vi "Teleop.vi"(10 "Match Info":T1={"Autonomous Elapsed Seconds"=0.0, "TeleOp Elapsed Seconds"=0.0, "Disabled Elapsed Seconds"=0.0, "Visited Autonomous"=FALSE, "Visited TeleOp"=FALSE, "Visited Disabled"=FALSE, "Autonomous Settings"={"Autonomous Style"=enum."Independent", "VI Refnum"=refnum}}, 11 "Call Context":T2) -> ()   [LabVIEW 2017]
doc: "This VI is called for each TeleOp packet received from the DS where the robot is not disabled. It is often used to read from the joysticks and update I/O or to update setpoints for timed control loops. It should complete and return within 20 milliseconds or it may miss DS packets."
uses:
  <vilib>/Rock Robotics/WPI/DriverStation/WPI_DriverStationDerivedRobotMode.ctl
  <vilib>/Rock Robotics/WPI/DriverStation/WPI_DriverStationMatch Info.ctl
  <vilib>/Rock Robotics/WPI/Utilities/WPI_GetSetVariantRefNum.vi
  <vilib>/Rock Robotics/Network Tables/NT Write Boolean Array.vi
  <vilib>/Rock Robotics/Network Tables/NT Write Numeric Array.vi
  <vilib>/Rock Robotics/Network Tables/NT Read Boolean.vi
  <vilib>/Rock Robotics/Network Tables/NT Read Number.vi
panel:
  out "Sample Slider 0":dbl(slide) scale=0.0..5.0
  out "Sample Boolean 1":bool
  out "Sample Boolean 0":bool
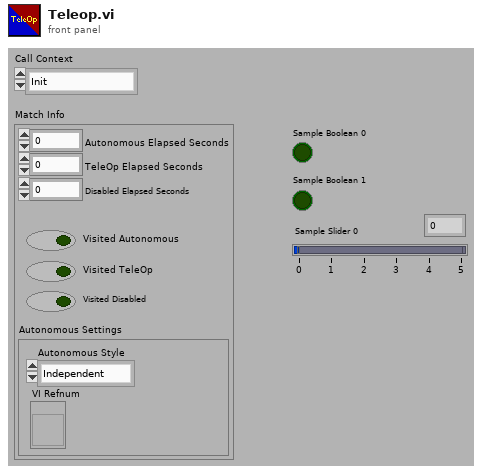
[diagram p1: front panel]
types:
  T1 = typedef "WPI_DriverStationMatch Info.ctl" = cluster{"Autonomous Elapsed Seconds":dbl, "TeleOp Elapsed Seconds":dbl, "Disabled Elapsed Seconds":dbl, "Visited Autonomous":bool, "Visited TeleOp":bool, "Visited Disabled":bool, "Autonomous Settings":cluster{"Autonomous Style":enum16{"Iterative", "Independent"}, "VI Refnum":refnum<vi>}}
  T2 = typedef "WPI_DriverStationDerivedRobotMode.ctl" = enum16{"Init", "Execute", "Stop"}
  T3 = typedef "WPI_JoystickDevRef.ctl" = cluster{"Device":T4}
  T4 = typedef "WPI_JoystickDeviceEnum.ctl" = enum16{"USB 0", "USB 1", "USB 2", "USB 3", "USB 4", "USB 5"}
  T5 = cluster{"Buttons[0]":bool, "Buttons[1]":bool, "Buttons[2]":bool, "Buttons[3]":bool, "Buttons[4]":bool, "Buttons[5]":bool, "Buttons[6]":bool, "Buttons[7]":bool, "Buttons[8]":bool}
  T6 = cluster{"Axes[0]":dbl, "Axes[1]":dbl, "Axes[2]":dbl, "Axes[3]":dbl, "Axes[4]":dbl, "Axes[5]":dbl, "Axes[6]":dbl, "Axes[7]":dbl, "Axes[8]":dbl}
  T7 = typedef "WPI_MotorControlDeviceRef.ctl" = cluster{"DeviceStatus":errorcluster, "Type":T8, "PWM":cluster{"PWM Channel":T9, "DeadBand":T10}, "CAN":cluster{"Device Number":u8, "SetOutput VI Ref":variant, "GetOutput VI Ref":variant, "Enable VI Ref":variant, "Disable VI Ref":variant, "Data":variant}, "Invert":bool, "DIO PWM":cluster{"PWM \"Enable\" Channel":T9, "DIOChannel":T11, "PWM Rate":dbl}}
  T8 = typedef "WPI_MotorControlType.ctl" = enum16{"PWM", "CAN", "DIO PWM"}
  T9 = typedef "FPGA_DIOPWMChannel.ctl" = enum8{"PWM 0", "PWM 1", "PWM 2", "PWM 3", "PWM 4", "PWM 5", "PWM 6", "PWM 7", "PWM 8", "PWM 9", "PWM MXP 0", "PWM MXP 1", "PWM MXP 2", "PWM MXP 3", "PWM MXP 4", "PWM MXP 5", "PWM MXP 6", "PWM MXP 7", "PWM MXP 8", "PWM MXP 9", "Invalid"}
  T10 = typedef "WPI_PWMDeadband.ctl" = cluster{"Name":string, "maxPositivePwm":i32, "minPositivePwm":i32, "centerPwm":i32, "maxNegativePwm":i32, "minNegativePwm":i32, "angularRange":u16}
  T11 = typedef "FPGA_DIOChannel.ctl" = enum8{"DIO 0", "DIO 1", "DIO 2", "DIO 3", "DIO 4", "DIO 5", "DIO 6", "DIO 7", "DIO 8", "DIO 9", "DIO MXP 0", "DIO MXP 1", "DIO MXP 2", "DIO MXP 3", "DIO MXP 4", "DIO MXP 5", "DIO MXP 6", "DIO MXP 7", "DIO MXP 8", "DIO MXP 9", "DIO MXP 10", "DIO MXP 11", "DIO MXP 12", "DIO MXP 13", "DIO MXP 14", "DIO MXP 15", "SPI Port CS1", "SPI Port CS2", "SPI Port CS3", "SPI Port MISO", "SPI Port MOSI", "Invalid"}
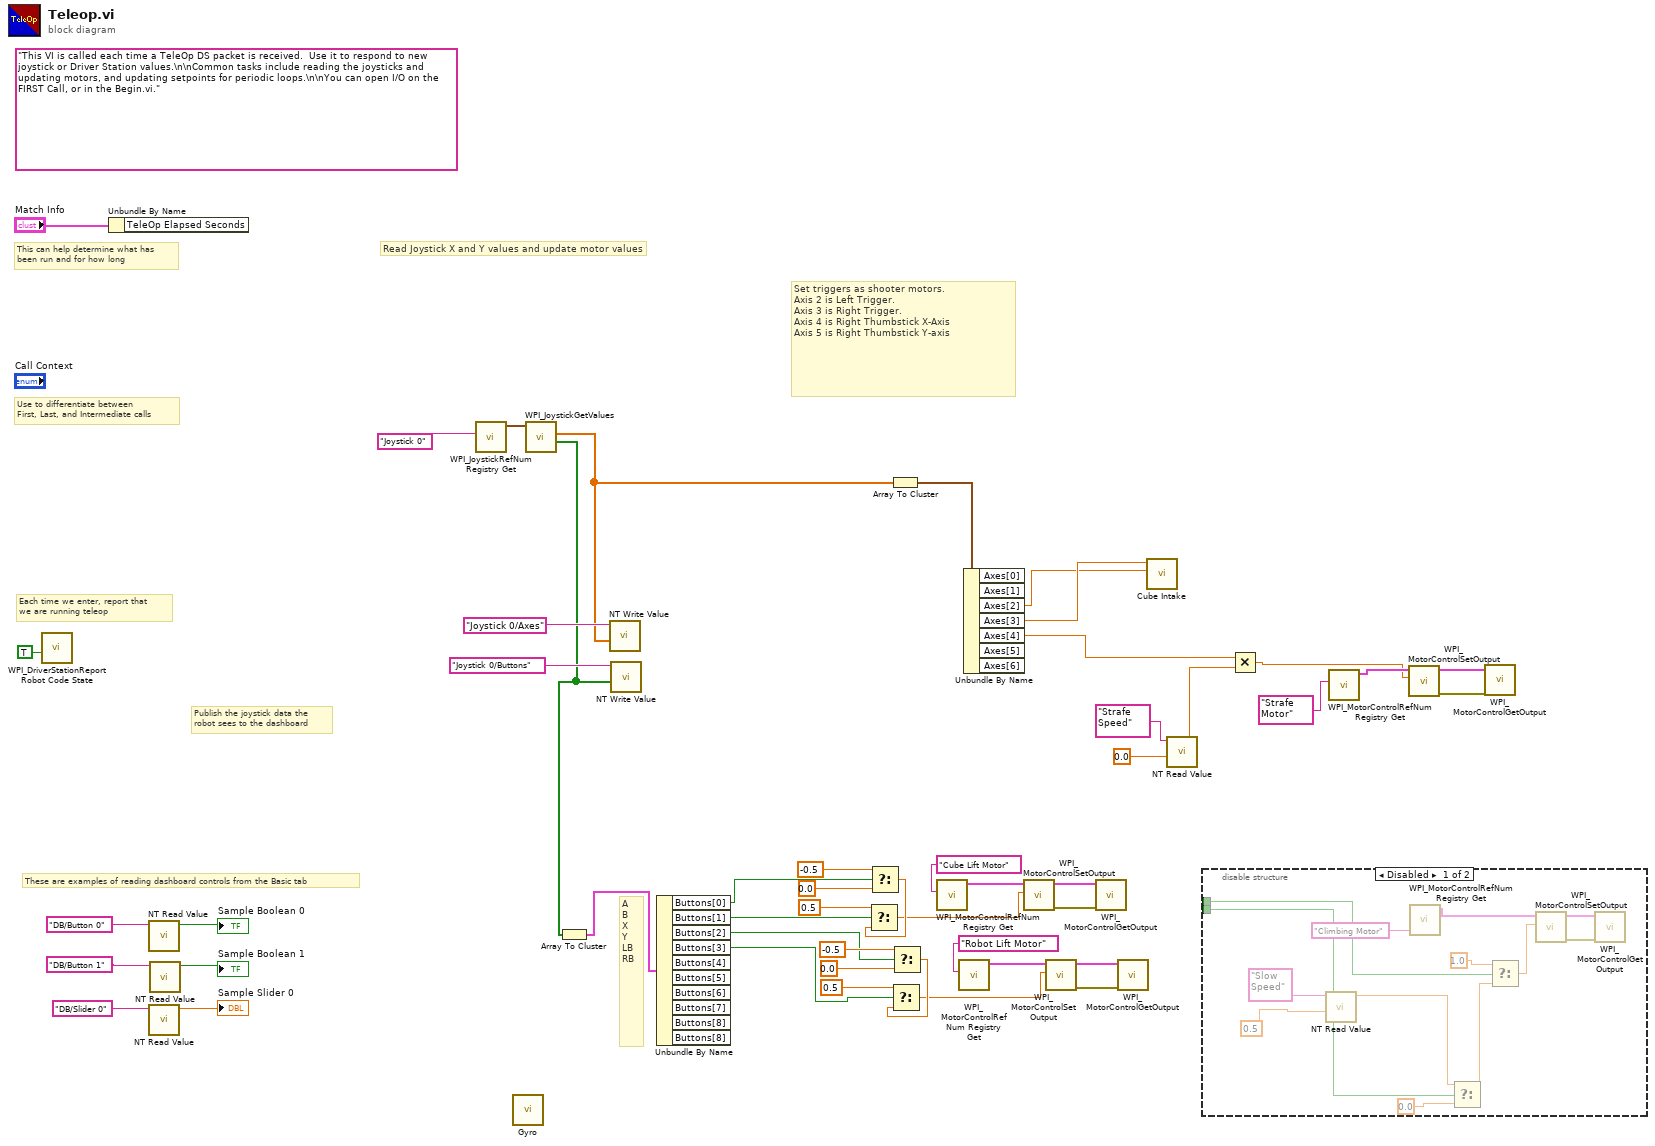
[diagram p0: block diagram]
diagram:
  (unwired) "This VI is called each time a TeleOp DS packet is received.  Use it to respond to new joystick or Driver Station values.\n\nCommon tasks include reading the joysticks and updating motors, and updating setpoints for periodic loops.\n\nYou can open I/O on the FIRST Call, or in the Begin.vi."
  # "Set triggers as shooter motors.  \nAxis 2 is Left Trigger.  \nAxis 3 is Right Trigger.\nAxis 4 is Right Thumbstick X-Axis\nAxis 5 is Right Thumbstick Y-axis"
  # "A\nB\nX\nY\nLB\nRB"
  # "These are examples of reading dashboard controls from the Basic tab"
  # "Publish the joystick data the\nrobot sees to the dashboard"
  # "Each time we enter, report that\nwe are running teleop"
  # "Use to differentiate between\nFirst, Last, and Intermediate calls"
  # "This can help determine what has\nbeen run and for how long"
  # "Read Joystick X and Y values and update motor values"
  n1 = call <vilib>:"WPI_DriverStationReport Robot Code State.vi"("TeleOp"=TRUE ("Autonomous")) -> ()  [unwired: 10 in, 1 out]
  n2 = Unbundle By Name("Match Info") -> ()  [unwired: 1 out]
  n3 = call-poly <vilib>:"NT Read Value.vi"("Name"="DB/Button 0" ("refnum name")) -> ("Boolean"=→"Sample Boolean 0":bool)  [unwired: 9 in, 1 out]
  n4 = call-poly <vilib>:"NT Read Value.vi"("Name"="DB/Slider 0" ("refnum name")) -> ("Numeric"=→"Sample Slider 0":dbl)  [unwired: 9 in, 1 out]
  n5 = call-poly <vilib>:"NT Read Value.vi"("Name"="DB/Button 1" ("refnum name")) -> ("Boolean"=→"Sample Boolean 1":bool)  [unwired: 9 in, 1 out]
  n6 = call <vilib>:"WPI_JoystickRefNum Registry Get.vi"("refnum name"="Joystick 0") -> ("JoystickDevRef"=w47:T3)  [unwired: 1 in, 9 out]
  n7 = call "Gyro.vi"() -> ()  [unwired: 12 in]
  n8 = call <vilib>:"WPI_JoystickGetValues.vi"("JoystickDevRef"=w47) -> ("Buttons"=w37:bool[], "Axes"=w35:dbl[])  [unwired: 6 in, 3 out]
  n9 = Array To Cluster(array=w37) -> (cluster=w18:T5)
  n10 = call-poly <vilib>:"NT Write Value.vi"("Numeric Array"=w35, "Name"="Joystick 0/Axes") -> ()  [unwired: 9 in, 1 out]
  n11 = call-poly <vilib>:"NT Write Value.vi"("Boolean Array"=w37, "Name"="Joystick 0/Buttons") -> ()  [unwired: 9 in, 1 out]
  n12 = Unbundle By Name(w18) -> ("Buttons[0]"=w15:bool, "Buttons[1]"=w17:bool, "Buttons[2]"=w2:bool, "Buttons[3]"=w1:bool)  [unwired: 6 out]
  n13 = Select(t=-0.5, s=w15, f=0.0) -> (s? t:f=w13:dbl)
  n14 = Select(t=0.5, s=w17, f=w13) -> (s? t:f=w12:dbl)
  n15 = Array To Cluster(array=w35) -> (cluster=w36:T6)
  n16 = Select(t=-0.5, s=w2, f=0.0) -> (s? t:f=w4:dbl)
  n17 = Select(t=0.5, s=w1, f=w4) -> (s? t:f=w3:dbl)
  n18 = call <vilib>:"WPI_MotorControlRefNum Registry Get.vi"("refnum name"="Cube Lift Motor") -> ("MotorControlDevRef"=w21:T7)  [unwired: 9 in, 1 out]
  n19 = call <vilib>:"WPI_MotorControlRefNum Registry Get.vi"("refnum name"="Robot Lift Motor") -> ("MotorControlDevRef"=w9:T7)  [unwired: 9 in, 1 out]
  n20 = Unbundle By Name(w36) -> ("Axes[2]"=w32:dbl, "Axes[3]"=w33:dbl, "Axes[4]"=w34:dbl)  [unwired: 4 out]
  n21 = call <vilib>:"WPI_MotorControlSetOutput.vi"("Output"=w12, "MotorControlDevRef"=w21) -> ("error out"=w23:errorcluster, "MotorControlDevRef"=w22:T7)  [unwired: 7 in, 1 out]
  n22 = call <vilib>:"WPI_MotorControlSetOutput.vi"("Output"=w3, "MotorControlDevRef"=w9) -> ("error out"=w11:errorcluster, "MotorControlDevRef"=w10:T7)  [unwired: 7 in, 1 out]
  n23 = call <vilib>:"WPI_MotorControlGetOutput.vi"("error in"=w23, "MotorControlDevRef"=w22) -> ()  [unwired: 7 in, 3 out]
  n24 = call <vilib>:"WPI_MotorControlGetOutput.vi"("error in"=w11, "MotorControlDevRef"=w10) -> ()  [unwired: 7 in, 3 out]
  n25 = call "Cube Intake.vi"("Axes[2]"=w32, "Axes[3]"=w33) -> ()  [unwired: 10 in]
  n26 = call-poly <vilib>:"NT Read Value.vi"("Default Value"=0.0, "Name"="Strafe Speed") -> ("Numeric"=w25:dbl)  [unwired: 8 in, 1 out]
  n27 = disable-structure shown="Disabled" {
    disable-tunnel: _ -> [w51 _]
    disable-tunnel: _ -> [w50 _]
    frame Disabled {
      n28 = call-poly <vilib>:"NT Read Value.vi"("Default Value"=0.5, "Name"="Slow Speed" ("refnum name")) -> ("Numeric"=w54:dbl)  [unwired: 8 in, 1 out]
      n29 = call <vilib>:"WPI_MotorControlRefNum Registry Get.vi"("refnum name"="Climbing Motor") -> ("MotorControlDevRef"=w53:T7)  [unwired: 9 in, 1 out]
      n30 = Select(t=w54, s=w50, f=0.0) -> (s? t:f=w57:dbl)
      n31 = Select(t=1.0, s=w51, f=w57) -> (s? t:f=w59:dbl)
      n32 = call <vilib>:"WPI_MotorControlSetOutput.vi"("Output"=w59, "MotorControlDevRef"=w53) -> ("error out"=w61:errorcluster, "MotorControlDevRef"=w62:T7)  [unwired: 7 in, 1 out]
      n33 = call <vilib>:"WPI_MotorControlGetOutput.vi"("error in"=w61, "MotorControlDevRef"=w62) -> ()  [unwired: 7 in, 3 out]
    }
    frame Enabled {
    }
  }
  n34 = Multiply(x=w34, y=w25) -> (x*y=w26:dbl)
  n35 = call <vilib>:"WPI_MotorControlRefNum Registry Get.vi"("refnum name"="Strafe Motor") -> ("MotorControlDevRef"=w30:T7)  [unwired: 9 in, 1 out]
  n36 = call <vilib>:"WPI_MotorControlSetOutput.vi"("Output"=w26, "MotorControlDevRef"=w30) -> ("error out"=w28:errorcluster, "MotorControlDevRef"=w29:T7)  [unwired: 7 in, 1 out]
  n37 = call <vilib>:"WPI_MotorControlGetOutput.vi"("error in"=w28, "MotorControlDevRef"=w29) -> ()  [unwired: 7 in, 3 out]
